vi "Acquire and Log Data.vi"(0 "TDMS Refnums in":refnum<k34>[](array[refnum]), 2 "rx config":T1={"rf enable 0"=TRUE, "rf config 0"={"antenna"="RX2", "frequency"=2000000000.0, "lo frequency"=-1.0, "level"=0.0}, "rf enable 1"=TRUE, "rf config 1"={"antenna"="RX2", "frequency"=2000000000.0, "lo frequency"=-1.0, "level"=0.0}, "transfer mode"=enum."Finite", "sample rate"=10000000.0, "start trigger"=enum."Immediate"} {"sample rate" format="%#.3pS/s"; "rf config 1"."level" format="%#_gdBm"; "rf config 1"."lo frequency" format="%#.3pHz"; "rf config 1"."frequency" format="%#.3pHz"; "rf config 0"."level" format="%#_gdBm"; "rf config 0"."lo frequency" format="%#.3pHz"; "rf config 0"."frequency" format="%#.3pHz"}, 5 "Refnum in":refnum<k20>[](array[refnum]), 7 "2 USRPs?":bool[](array[boolean]), 9 "Data Queue in":refnum<queue>, 11 "error in (no error)":errorcluster, 12 "Samples per Read":u32=1024000 format="%.3p", 13 "Previewed Channel":T3) -> (4 "TDMS Refnums out":refnum<k34>[](array[refnum]), 6 "Refnum out":refnum<k20>[](array[refnum]), 10 "Array":bool[](array[boolean]), 15 "error out":errorcluster)   [LabVIEW 2016]
uses:
  TDMS Raw to Channels/Previewed Channel - Enum.ctl
  TypeDefs/Rx Config.ctl
  2954/SubVIs/Start Trigger.ctl
  6592R/SubVIs/Aurora Stream (NI 6592R) (Host).lvlib
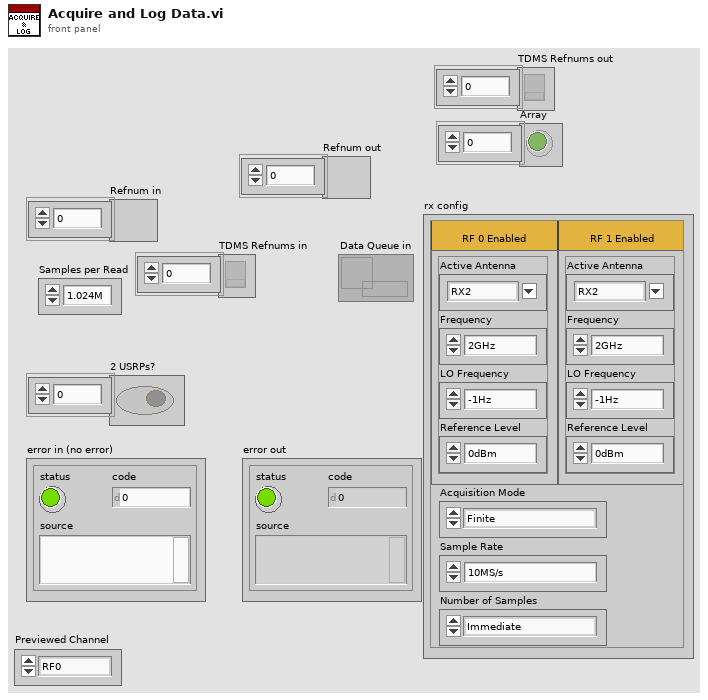
[diagram p1: front panel]
types:
  T1 = typedef "Rx Config.ctl" = cluster{"rf enable 0":bool, "rf config 0":cluster{"antenna":string, "frequency":dbl, "lo frequency":dbl, "level":dbl}, "rf enable 1":bool, "rf config 1":cluster{"antenna":string, "frequency":dbl, "lo frequency":dbl, "level":dbl}, "transfer mode":enum16{"Finite", "Continuous"}, "sample rate":dbl, "start trigger":T2}
  T2 = typedef "Start Trigger.ctl" = enum8{"Software", "Digital Edge", "Rx Start Trigger", "Tx Start Trigger", "Immediate", "Future Time Event"}
  T3 = typedef "Previewed Channel - Enum.ctl" = enum16{"RF0", "RF1"}
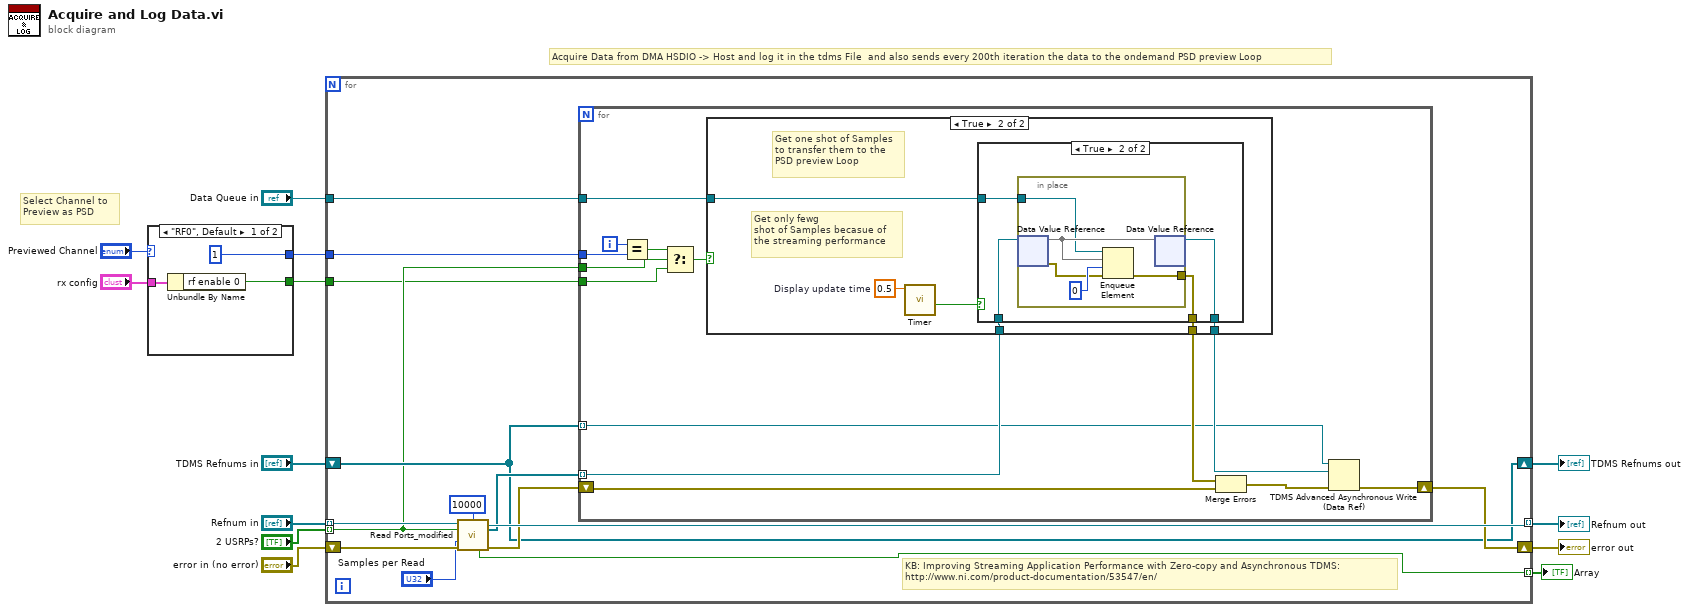
[diagram p0: block diagram]
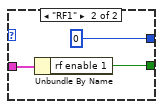
[diagram p2: hidden frame]
diagram:
  # "Select Channel to \nPreview as PSD"
  # "Acquire Data from DMA HSDIO -> Host and log it in the tdms File  and also sends every 200th iteration the data to the ondemand PSD preview Loop"
  n1 = case shown="\"RF0\", Default" "Previewed Channel" {
    tunnel: [1 ("y") 0 ("y")] -> w6
    tunnel: "rx config" -> [w14 w18]
    tunnel: [w15 w17] -> w1
    frame "RF0", Default {
      n2 = Unbundle By Name(w14) -> ("rf enable 0"=w15:bool)
    }
    frame "RF1" {
      n3 = Unbundle By Name(w18) -> ("rf enable 1"=w17:bool)
    }
  }
  n4 = for {
    tunnel: "Refnum in" -> [w32] mode=indexing
    shift-right: [w26] -> w13
    shift-left: "error in (no error)" -> [w33]
    tunnel: "2 USRPs?" -> [w21] mode=indexing
    tunnel: [w30] -> w10 mode=indexing
    tunnel: "Data Queue in" -> [w25]
    tunnel: w6 -> [w24]
    shift-right: [w23] -> w4
    shift-left: "TDMS Refnums in" -> [w23]
    tunnel: [w22] -> w3 mode=indexing
    tunnel: w1 -> [w20]
    # "KB: Improving Streaming Application Performance with Zero-copy and Asynchronous TDMS:\nhttp://www.ni.com/product-documentation/53547/en/"
    n5 = call "Read Ports_modified.vi"("Refnum in"=w32, "timeout (ms)"=10000 ("Timeout (ms)"), "2 Ports"=w21, "number of elements"="Samples per Read", "error in"=w33) -> ("Refnum out"=w30:refnum<k20>, "Read Region References"=w28:refnum<data-value>[], "Data Valid"=w22:bool, "error out"=w27:errorcluster)  [unwired: 5 in, 2 out]
    n6 = for {
      tunnel: w28 -> [w45] mode=indexing
      shift-right: [w47] -> w26
      shift-left: w27 -> [w43]
      tunnel: w25 -> [w46]
      tunnel: w24 -> [w44]
      tunnel: w23 -> [w39] mode=indexing
      tunnel: w21 -> [w36]
      tunnel: w20 -> [w34]
      i -> [w38]
      n7 = Equal?(x=w38, y=w44) -> (x = y?=w35:bool)
      n8 = Select(t=w35, s=w36, f=w34) -> (s? t:f=w37:bool)
      n9 = case shown="True" w37 {
        tunnel: w46 -> [_ w54]
        tunnel: w45 -> [w48 w53]
        tunnel: [w48 w52] -> w42
        tunnel: [_ w51] -> w40
        frame False {
        }
        frame True {
          w49 = 0.5  # Display update time
          # "Get only fewg\nshot of Samples becasue of \nthe streaming performance"
          # "Get one shot of Samples\nto transfer them to the \nPSD preview Loop"
          n10 = call "Timer.vi"("Set Time [s]"=w49) -> ("Time elapsed!"=w50:bool)  [unwired: 9 in, 1 out]
          n11 = case shown="True" w50 {
            tunnel: w54 -> [_ w59]
            tunnel: w53 -> [w55 w58]
            tunnel: [w55 w57] -> w52
            tunnel: [_ w56] -> w51
            frame False {
            }
            frame True {
              n12 = in-place {
                in-place-border: w59 -> [w63]
                in-place-border: [w60] -> w56
                n13 = in-place-dvr #1(w58) -> (w64:u64[], w61:errorcluster)
                n14 = Enqueue Element(queue=w63, element=w64, timeout in ms (-1)=0, error in (no error)=w61) -> (error out=w60:errorcluster)  [unwired: 2 out]
                n15 = in-place-dvr #1(w64) -> (w57:refnum<data-value>)  [unwired: 1 out]
              }
            }
          }
        }
      }
      n16 = Merge Errors(w40, w43) -> (w41:errorcluster)
      n17 = TDMS Advanced Asynchronous Write (Data Ref)(8:w41, 10:w42, 11:w39) -> (0:w47:errorcluster)  [unwired: 1 in, 1 out]
    }
  }
  "error out" <- w13
  "Refnum out" <- w10
  "TDMS Refnums out" <- w4
  "Array" <- w3
